vi "Property Nodes - Fill Tank Color.vi"() -> ()   [LabVIEW 2014]
panel:
  in  "Stop Button":bool
  out "Tank":dbl(slide) scale=0.0..10.0
  in  "Alarm Level":dbl(slide) scale=0.0..10.0
  in  "Fill Level":dbl(slide) scale=0.0..10.0
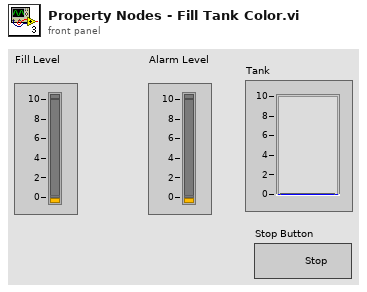
[diagram p1: front panel]
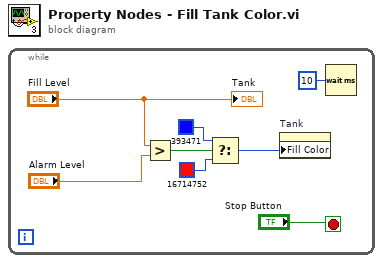
[diagram p0: block diagram]
diagram:
  n1 = while {
    stop <- "Stop Button" stop-if-true
    n2 = Greater?(x="Fill Level", y="Alarm Level") -> (0:w3:bool)
    n3 = Select(t=u32 393471, s=w3, f=u32 16714752) -> (s? t:f=w1:u32)
    n4 = property on="Tank" class="Slide (strict)"("Fill Color"=w1) -> ()  [unwired: 2 in, 2 out]
    n5 = Wait (ms)(milliseconds to wait=u32 10) -> ()  [unwired: 1 out]
    "Tank" <- "Fill Level"
  }
